vi "pointToLine.vi"(8 "error in (no error)":errorcluster, 10 "Line":T1 {"Point 2"."Y" format="%.2f"; "Point 2"."X" format="%.2f"; "Point 1"."Y" format="%.2f"; "Point 1"."X" format="%.2f"}, 11 "Point":cluster{"X":sgl, "Y":sgl}) -> (0 "error out":errorcluster, 2 "distance":dbl, 3 "Line":T1)   [LabVIEW 2019]
doc: "Computes the perpendicular distance between a line and a point."
uses:
  <vilib>/vision/NI_Vision_Development_Module.lvlib
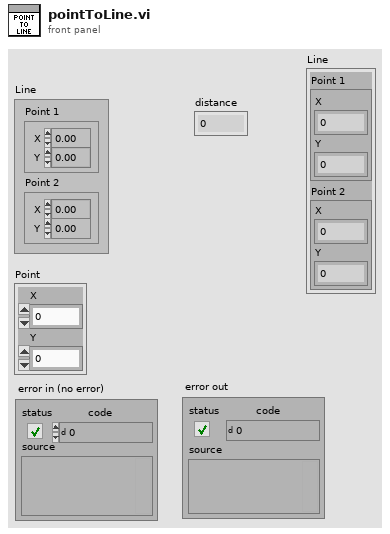
[diagram p1: front panel]
types:
  T1 = cluster{"Point 1":cluster{"X":sgl, "Y":sgl}, "Point 2":cluster{"X":sgl, "Y":sgl}}
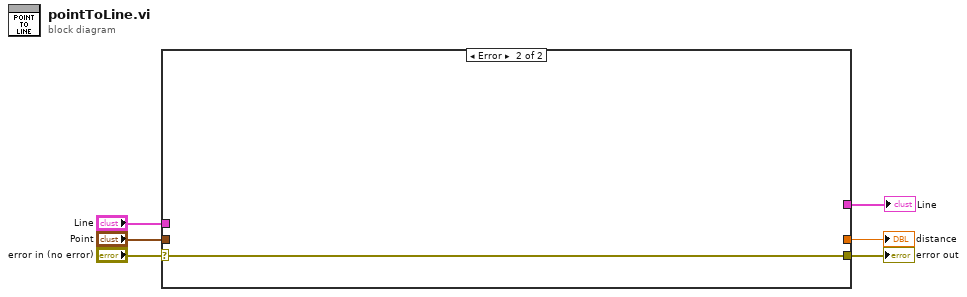
[diagram p0: block diagram]
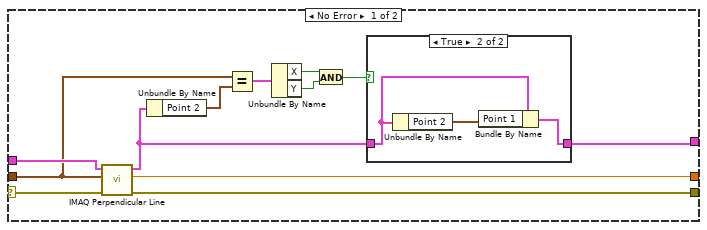
[diagram p2: hidden frame]
diagram:
  n1 = case shown="Error" "error in (no error)" {
    selector: "error in (no error)" -> [w17 w23]
    tunnel: [w18 w23] -> w5
    tunnel: [w16 _] -> w4
    tunnel: "Point" -> [w14 _]
    tunnel: "Line" -> [w15 _]
    tunnel: [w9 _] -> w1
    frame No Error {
      n2 = call "IMAQ Perpendicular Line"("error in (no error)"=w17, "Point"=w14, "Line"=w15) -> ("error out"=w18:errorcluster, "Distance"=w16:dbl, "Perpendicular Line"=w7:T1)  [unwired: 6 in]
      n3 = Unbundle By Name(w7) -> ("Point 2"=w13:cluster{"X":sgl, "Y":sgl})
      n4 = Equal?(x=w14, y=w13) -> (x = y?=w12:cluster{"X":bool, "Y":bool})
      n5 = Unbundle By Name(w12) -> ("X"=w11:bool, "Y"=w10:bool)
      n6 = And(x=w11, y=w10) -> (x .and. y?=w8:bool)
      n7 = case shown="True" w8 {
        tunnel: w7 -> [w19 w22]
        tunnel: [w19 w20] -> w9
        frame False {
        }
        frame True {
          n8 = Unbundle By Name(w22) -> ("Point 2"=w21:cluster{"X":sgl, "Y":sgl})
          n9 = Bundle By Name(cluster=w22, "Point 1"=w21) -> (w20:T1)
        }
      }
    }
    frame Error {
    }
  }
  "error out" <- w5
  "distance" <- w4
  "Line" <- w1
